vi "Close.vi"(8 "Error In":errorcluster, 11 "Channel In":refnum<class "Channel.lvclass">) -> (0 "Error Out":errorcluster, 3 "Channel Out":refnum<class "Channel.lvclass">)   [LabVIEW 2018, in "Toolkit.lvlib" / "Channel.lvclass"]
uses:
  Channel.lvclass
  Channel.lvclass/Channel.ctl
  Session/Session.lvclass/Session.ctl
  SSH/SSH.lvclass/SSH.ctl
  Session/Session.lvclass
  Toolkit.lvlib
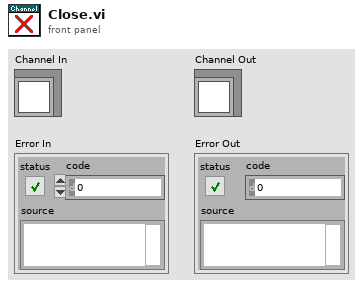
[diagram p1: front panel]
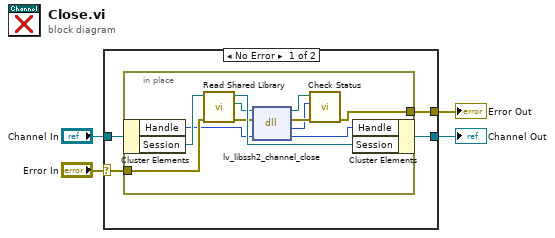
[diagram p0: block diagram]
diagram:
  n1 = case shown="No Error" "Error In" {
    selector: "Error In" -> [w6 w21]
    tunnel: [w5 w21] -> w3
    tunnel: "Channel In" -> [w8 w20]
    tunnel: [w7 w20] -> w1
    frame No Error {
      n2 = in-place {
        in-place-border: w6 -> [w15]
        in-place-border: [w11] -> w5
        n3 = in-place-cluster #1(w8) -> ("Handle"=w10:u64, "Session"=w19:refnum<class "Session.lvclass">)
        n4 = call "Read Shared Library.vi"("Error In"=w15, "Session In"=w19) -> ("Erorr Out"=w16:errorcluster, "libssh2lv Shared Library"=w17:path, "Session Out"=w18:refnum<class "Session.lvclass">)  [unwired: 7 in]
        n5 = dll-call lib="libssh2lv.*" fn="lv_libssh2_channel_close"(path in=w17, error in=w16, "handle"=w10) -> (path out=w13:path, error out=w14:errorcluster, "status"=w12:i32, "handle"=w9:u64)  [unwired: 1 in]
        n6 = call "Check Status.vi"("Error In"=w14, "Status"=w12, "lv-libssh2 Shared Library In"=w13) -> ("Error Out"=w11:errorcluster)  [unwired: 7 in, 1 out]
        n7 = in-place-cluster #1("Handle"=w9, "Session"=w18) -> (w7:refnum<class "Channel.lvclass">)
      }
    }
    frame Error {
    }
  }
  "Error Out" <- w3
  "Channel Out" <- w1
